vi "GetVisaResourceNameReference.vi"(8 "error in":errorcluster, 11 "VisaResourceName in":refnum<class "VisaResourceName.lvclass">) -> (0 "error out":errorcluster, 1 "Visa Resource reference":refnum<vi>, 3 "VisaResourceName out":refnum<class "VisaResourceName.lvclass">)   [LabVIEW 2014, in "Raspberry Pi Compatible Compiler for LabVIEW.lvlib" / "VisaResourceName.lvclass"]
uses:
  VisaResourceName.lvclass
  Generic/Generic.lvclass
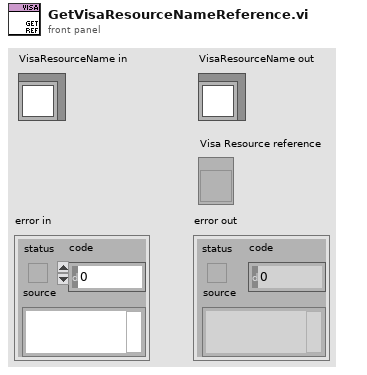
[diagram p1: front panel]
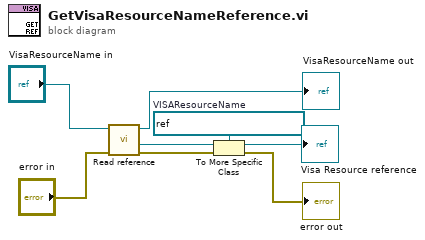
[diagram p0: block diagram]
diagram:
  w4 = refnum<vi> refnum  # VISAResourceName
  n1 = call "Read reference.vi"("error in"="error in", "GObject in"="VisaResourceName in") -> ("error out"=w5:errorcluster, "reference"=w6:refnum<vi>, "GObject out"=→"VisaResourceName out":refnum<class "VisaResourceName.lvclass">)  [unwired: 5 in]
  n2 = To More Specific Class(target class=w4, reference=w6, error in=w5) -> (specific class reference=→"Visa Resource reference":refnum<vi>, error out=→"error out":errorcluster)
